vi "GetTerminalOwner__slk_mt.vi"(8 "error in (no error)":errorcluster, 11 "terminal refnum in":refnum<vi>) -> (0 "error out":errorcluster, 3 "owner refnum out":refnum<vi>)   [LabVIEW 2013, in "Lazyboots Menu Tool.lvlib"]
doc: "Returns the owner of a terminal, such as shift register, tunnel and so on.\n\n<b>NOTE</b>: If the terminal is control terminal, it will return itself."
uses:
  Library/Lazyboots Menu Tool.lvlib
panel:
  # "GetTerminalOwner__slk_mt.vi\nReturns the owner of a terminal, such as shift register, tunnel and so on.\n\nNOTICE -- YOU MUST LEAVE THIS NOTICE IN PLACE.\n\nCopyright (c) 2011, LIANG LIU Shawn.Liu.cn@gmail.com\nAll rights reserved.\n\nRedistribution and use in source and binary forms, with or without modification, are permitted provided that the following conditions are met:\n-Redistributions of source code must retain the above copyright notice, this list of conditions and the following disclaimer.\n-Redistributions in binary form must reproduce the above copyright notice, this list of conditions and the following disclaimer in the documentation and/or other materials provided with the distribution.\n-Neither the name of the eLp nor the names of its contributors may be used to endorse or promote products derived from this software without specific prior written permission.\n\nTHIS SOFTWARE IS PROVIDED BY THE COPYRIGHT HOLDERS AND CONTRIBUTORS \"AS IS\" AND ANY EXPRESS OR IMPLIED WARRANTIES, INCLUDING, BUT NOT LIMITED TO, THE IMPLIED WARRANTIES OF MERCHANTABILITY AND FITNESS FOR A PARTICULAR PURPOSE ARE DISCLAIMED. IN NO EVENT SHALL THE COPYRIGHT HOLDER OR CONTRIBUTORS BE LIABLE FOR ANY DIRECT, INDIRECT, INCIDENTAL, SPECIAL, EXEMPLARY, OR CONSEQUENTIAL DAMAGES (INCLUDING, BUT NOT LIMITED TO, PROCUREMENT OF SUBSTITUTE GOODS OR SERVICES; LOSS OF USE, DATA, OR PROFITS; OR BUSINESS INTERRUPTION) HOWEVER CAUSED AND ON ANY THEORY OF LIABILITY, WHETHER IN CONTRACT, STRICT LIABILITY, OR TORT (INCLUDING NEGLIGENCE OR OTHERWISE) ARISING IN ANY WAY OUT OF THE USE OF THIS SOFTWARE, EVEN IF ADVISED OF THE POSSIBILITY OF SUCH DAMAGE."
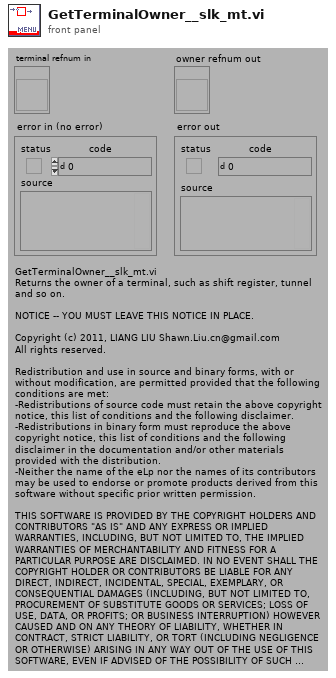
[diagram p1: front panel]
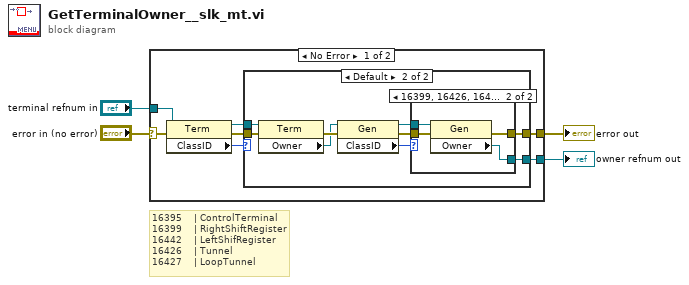
[diagram p0: block diagram]
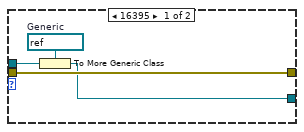
[diagram p2: hidden frame]
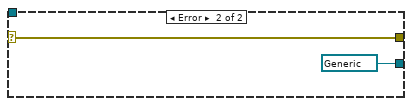
[diagram p4: hidden frame]
diagram:
  # "16395    | ControlTerminal\n16399    | RightShiftRegister\n16442    | LeftShifRegister\n16426    | Tunnel\n16427    | LoopTunnel"
  n1 = case shown="No Error" "error in (no error)" {
    selector: "error in (no error)" -> [w5 w32]
    tunnel: "terminal refnum in" -> [w6 _]
    tunnel: [w8 refnum<vi> refnum ("Owner")] -> w3
    tunnel: [w7 w32] -> w2
    frame No Error {
      n2 = property on="Property Node" class="Term"(reference=w6, error in=w5) -> (reference out=w10:refnum<vi>, error out=w11:errorcluster, "ClassID"=w9:u32)
      n3 = case shown="Default" w9 {
        tunnel: w11 -> [w14 w24]
        tunnel: [w14 w19] -> w7
        tunnel: [w13 w18] -> w8
        tunnel: w10 -> [w15 w16]
        frame 16395 {
          w12 = refnum<vi> refnum  # Generic
          n4 = To More Generic Class(target class=w12, reference=w15) -> (generic class reference=w13:refnum<vi>)
        }
        frame Default {
          n5 = property class="Term"(reference=w16, error in=w24) -> (error out=w20:errorcluster, "Owner"=w17:refnum<vi>)  [unwired: 1 out]
          n6 = property on="Property Node" class="Gen"(reference=w17, error in=w20) -> (reference out=w22:refnum<vi>, error out=w23:errorcluster, "ClassID"=w21:u32)
          n7 = case shown="16399, 16426, 16427, 16442" w21 {
            tunnel: w22 -> [w26 w30]
            tunnel: [w26 w29] -> w18
            tunnel: w23 -> [w25 w28]
            tunnel: [w25 w27] -> w19
            frame Default {
            }
            frame 16399, 16426, 16427, 16442 {
              n8 = property class="Gen"(reference=w30, error in=w28) -> (error out=w27:errorcluster, "Owner"=w29:refnum<vi>)  [unwired: 1 out]
            }
          }
        }
      }
    }
    frame Error {
    }
  }
  "owner refnum out" <- w3
  "error out" <- w2
